vi "init.vi"(8 "error in (no error)":errorcluster, 11 "IDE simple in":refnum<class "Main Panel.lvclass">) -> (0 "error out":errorcluster, 3 "IDE simple out":refnum<class "Main Panel.lvclass">)   [LabVIEW 2018, in "Main Panel.lvlib" / "Main Panel.lvclass"]
uses:
  Main Panel.lvclass
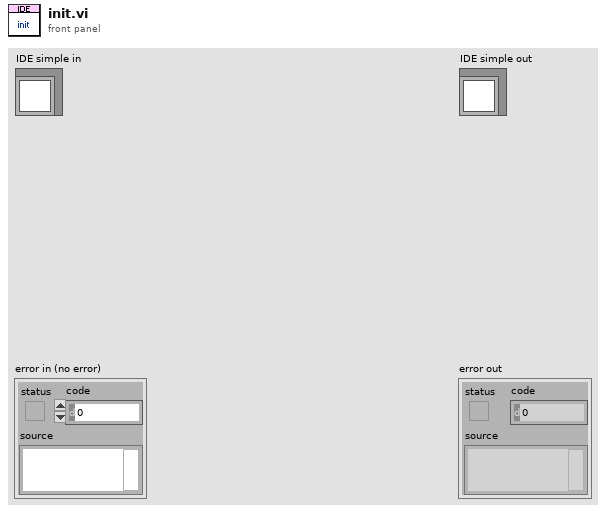
[diagram p1: front panel]
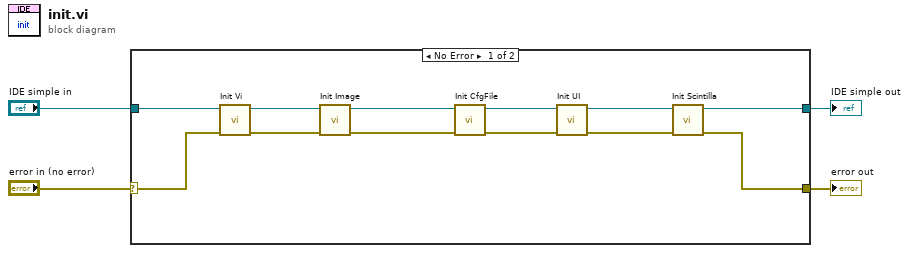
[diagram p0: block diagram]
diagram:
  n1 = case shown="No Error" "error in (no error)" {
    selector: "error in (no error)" -> [w15 w18]
    tunnel: [w13 w18] -> w3
    tunnel: [w14 w17] -> w1
    tunnel: "IDE simple in" -> [w16 w17]
    frame No Error {
      n2 = call "Init Vi.vi"("error in (no error)"=w15, "IDE simple in"=w16) -> ("error out"=w11:errorcluster, "IDE simple out"=w12:refnum<class "Main Panel.lvclass">)  [unwired: 8 in]
      n3 = call "Init Image.vi"("error in (no error)"=w11, "LF2R IDE in"=w12) -> ("error out"=w9:errorcluster, "LF2R IDE out"=w10:refnum<class "Main Panel.lvclass">)  [unwired: 8 in]
      n4 = call "Init CfgFile.vi"("error in (no error)"=w9, "LF2R IDE in"=w10) -> ("error out"=w7:errorcluster, "LF2R IDE out"=w8:refnum<class "Main Panel.lvclass">)  [unwired: 8 in]
      n5 = call "Init UI.vi"("error in (no error)"=w7, "LF2R IDE in"=w8) -> ("error out"=w5:errorcluster, "LF2R IDE out"=w6:refnum<class "Main Panel.lvclass">)  [unwired: 8 in]
      n6 = call "Init Scintilla.vi"("error in (no error)"=w5, "LF2R IDE in"=w6) -> ("error out"=w13:errorcluster, "LF2R IDE out"=w14:refnum<class "Main Panel.lvclass">)  [unwired: 8 in]
    }
    frame Error {
    }
  }
  "error out" <- w3
  "IDE simple out" <- w1
